vi "GetSavingPath.vi"(8 "error in":errorcluster, 10 "ArgIndex (0)":i32, 11 "Args":string[](array[string])) -> (0 "error out":errorcluster, 2 "SavingPath[String]":string, 3 "SavingPath":path)   [LabVIEW 2020]
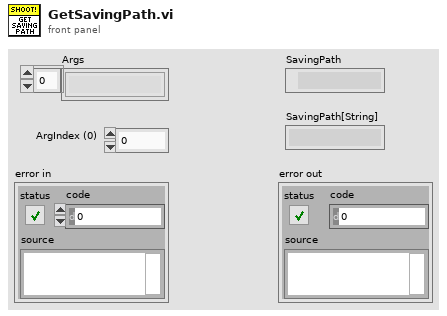
[diagram p1: front panel]
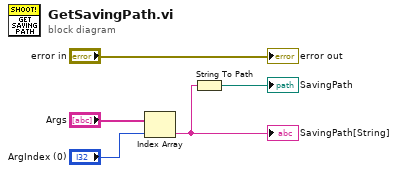
[diagram p0: block diagram]
diagram:
  n1 = Index Array(array="Args", index="ArgIndex (0)") -> (element=w4:string)
  "SavingPath[String]" <- w4
  n2 = String To Path(string=w4) -> (path=→"SavingPath":path)
  "error out" <- "error in"
